vi "strip settings file.vi"(0 "strip array in":string[][](array[string])) -> (1 "time array":timestamp[](array[timestamp]), 2 "settings array out":string[][](array[string]), 3 "timer graph":cluster{cluster{timestamp, dbl}[]}[](graph), 4 "Xscalemax":dbl, 5 "cursor position":dbl, 6 "Xscle min":dbl)   [LabVIEW 2018]
panel:
  out "sec":string
  out "m":string
  out "h":string
  out "DeltaT?":bool
  out "subarray":string[](array[string])
  out "concatenated time string 2":string
  out "function 2":string
  out "cluster 2":T1
  out "strip array 3":string[](array[string])
  out "array of clusters 2":cluster{cluster{timestamp, dbl}[]}[](array[cluster])
  out "cluster":T1
  out "plight":i32=1
  out "mlight":i32=1
  out "function":string
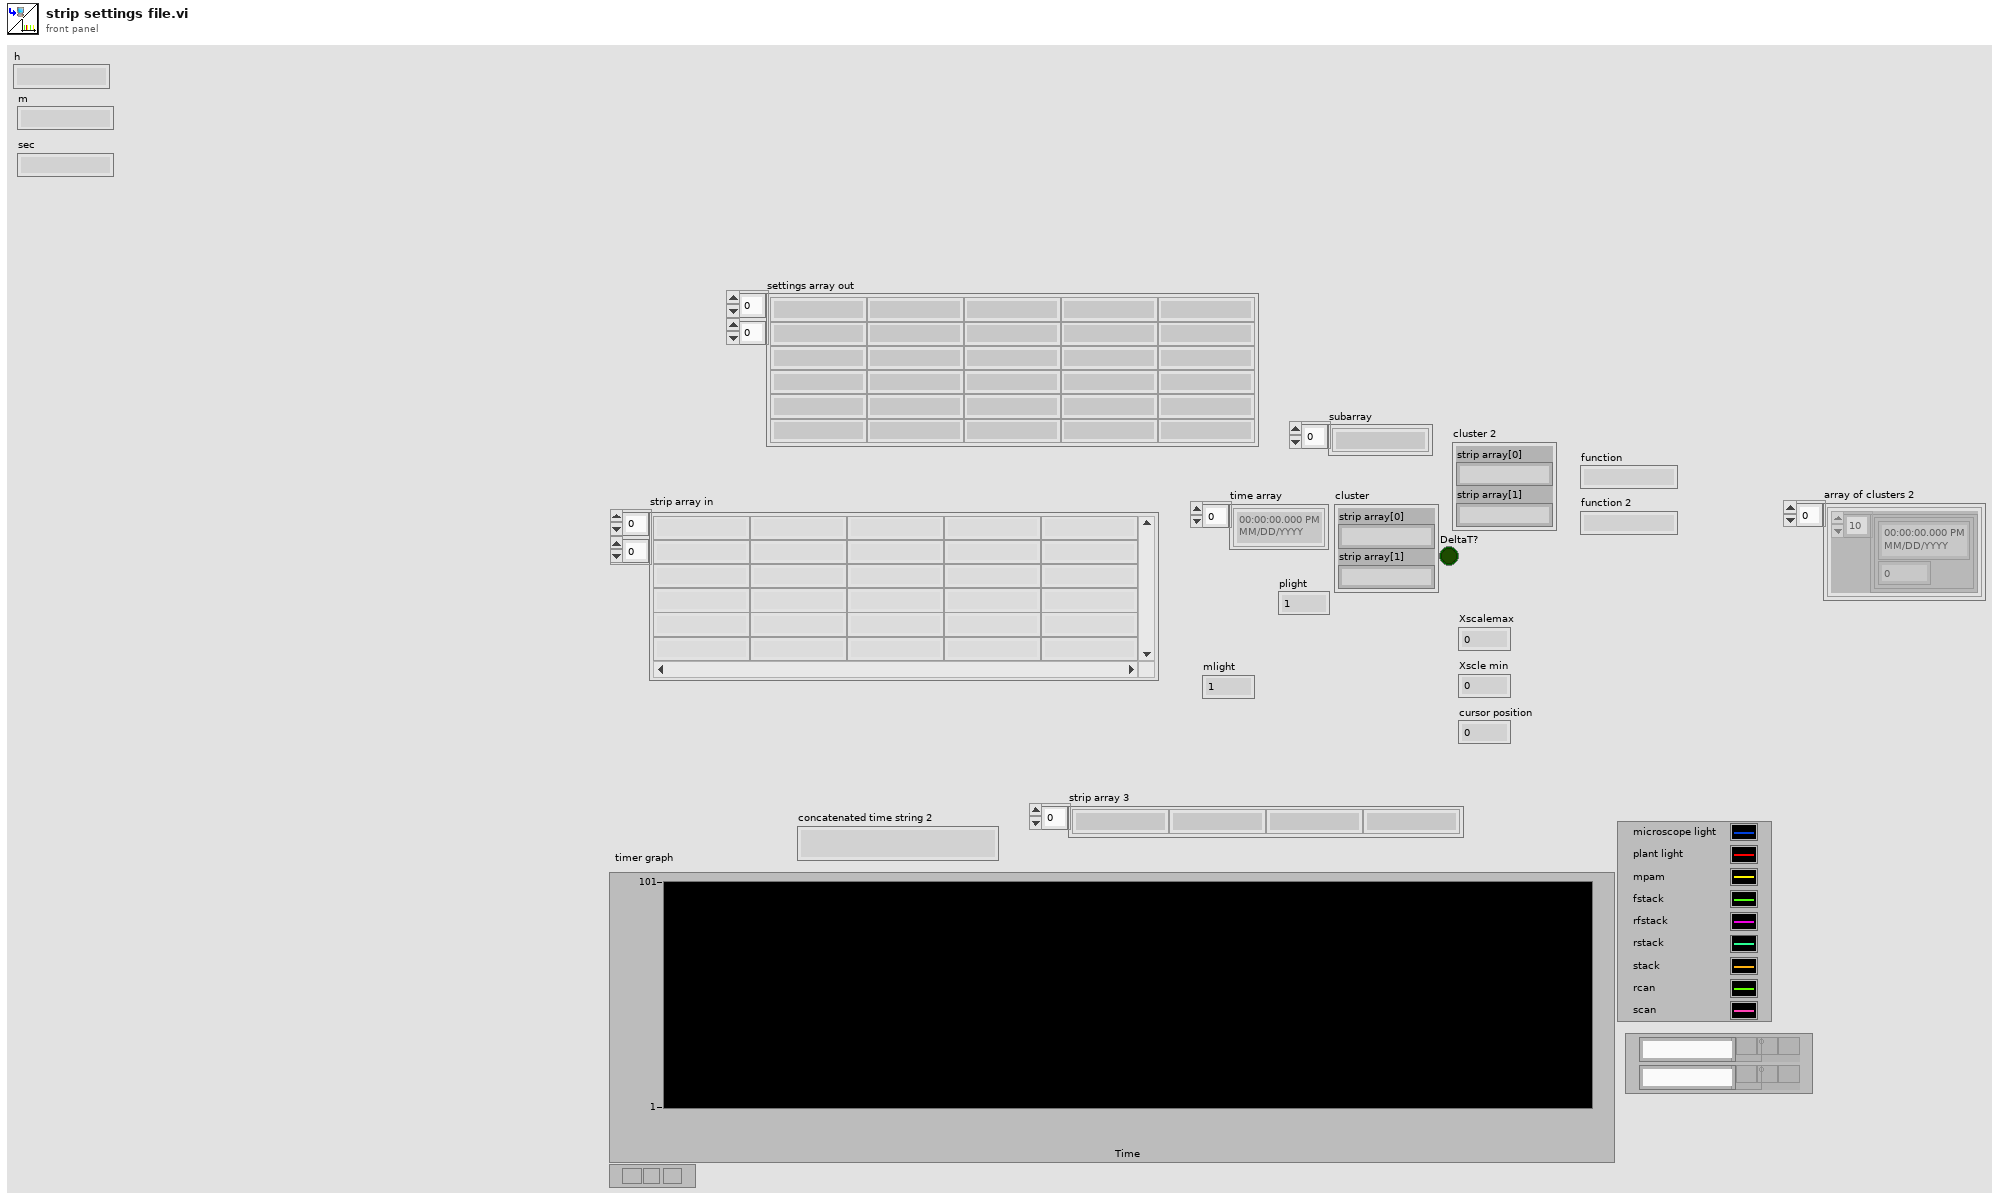
[diagram p1: front panel]
types:
  T1 = cluster{"strip array[0]":string, "strip array[1]":string}
  T2 = cluster{"strip array in[0]":string, "strip array in[1]":string}
  T3 = cluster{"strip array in[0]":string, "strip array in[1]":string, "strip array in[2]":string, "strip array in[3]":string, "strip array in[4]":string, "strip array in[5]":string}
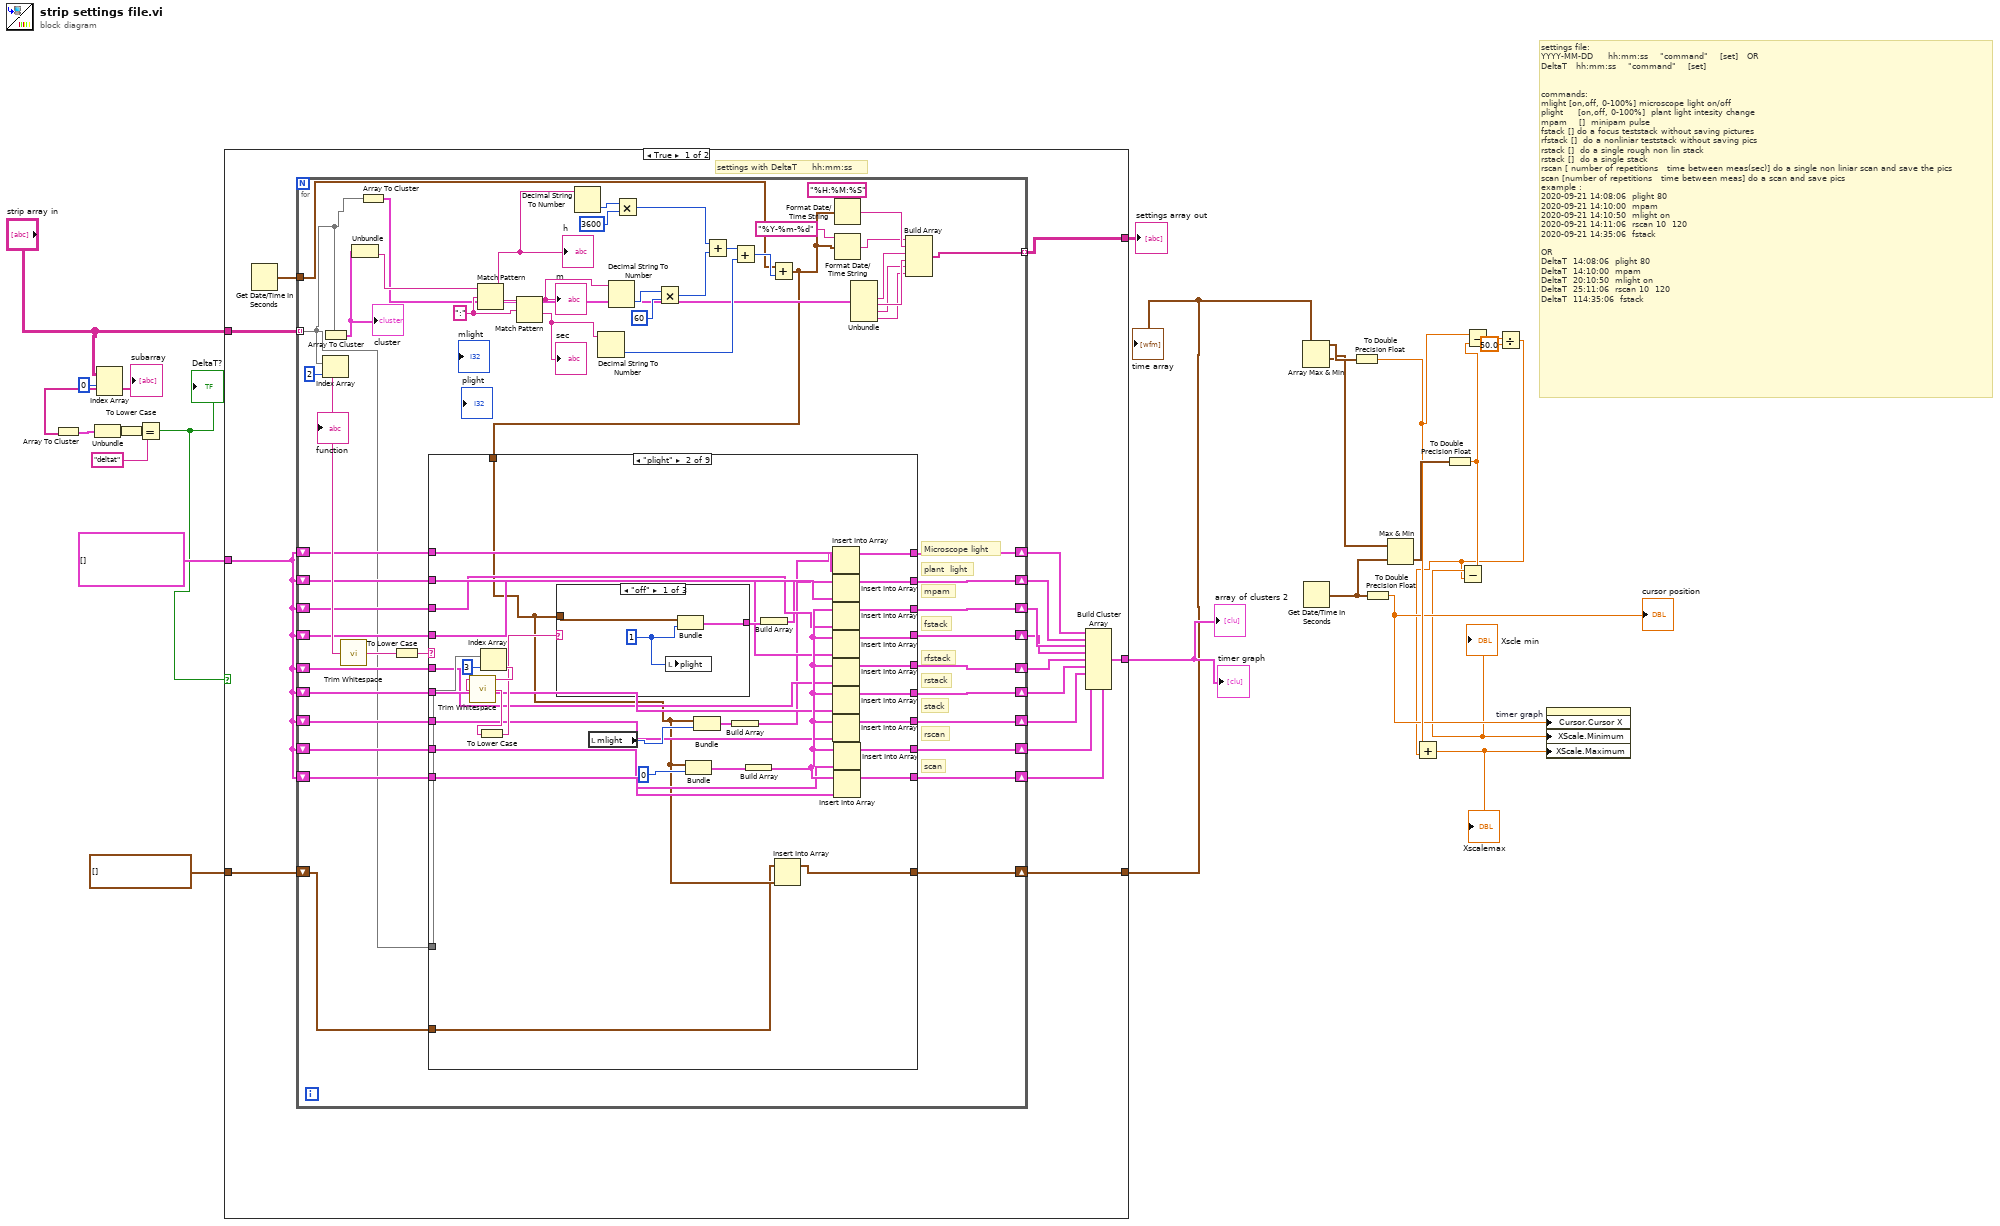
[diagram p0: block diagram]
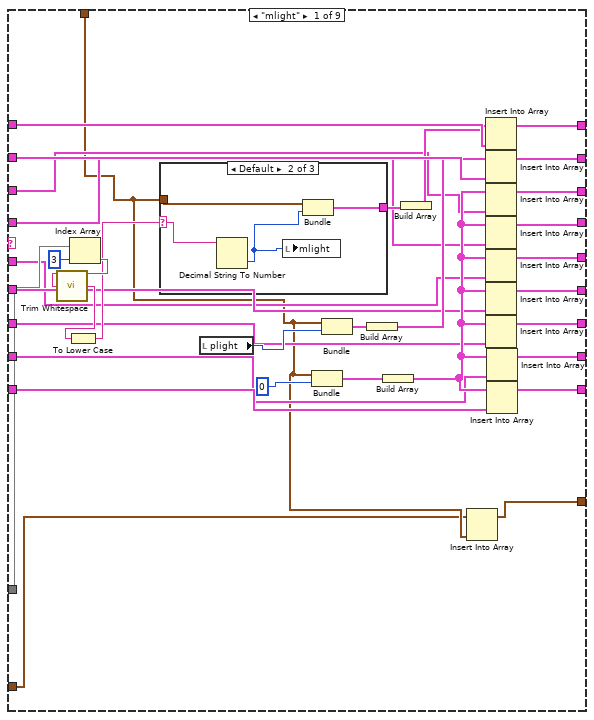
[diagram p2: hidden frame]
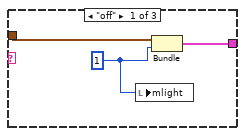
[diagram p3: hidden frame]
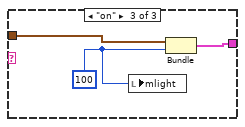
[diagram p4: hidden frame]
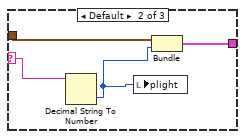
[diagram p5: hidden frame]
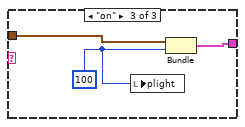
[diagram p6: hidden frame]
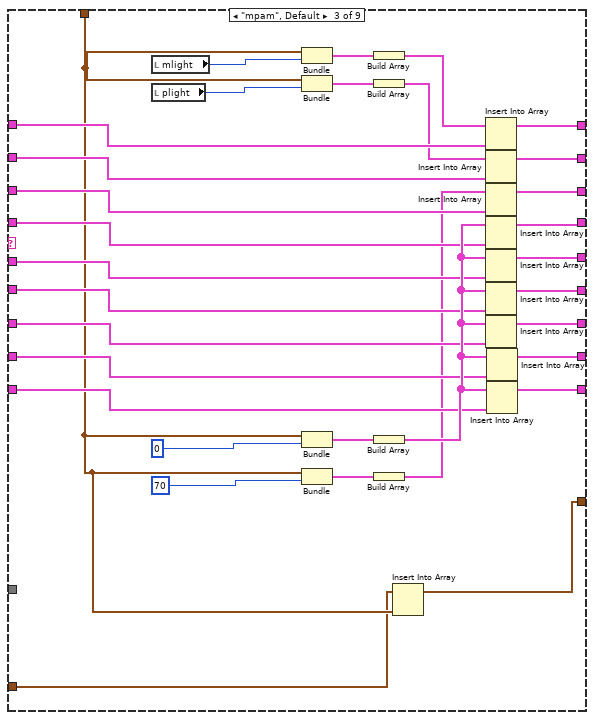
[diagram p7: hidden frame]
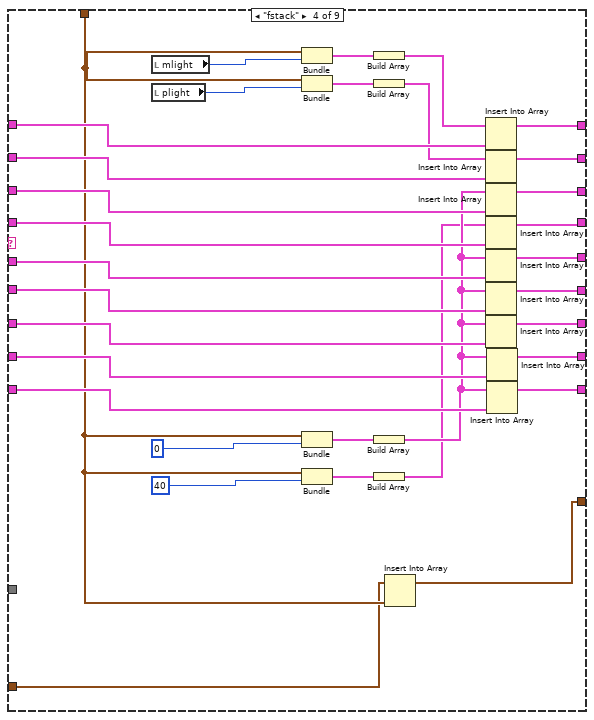
[diagram p8: hidden frame]
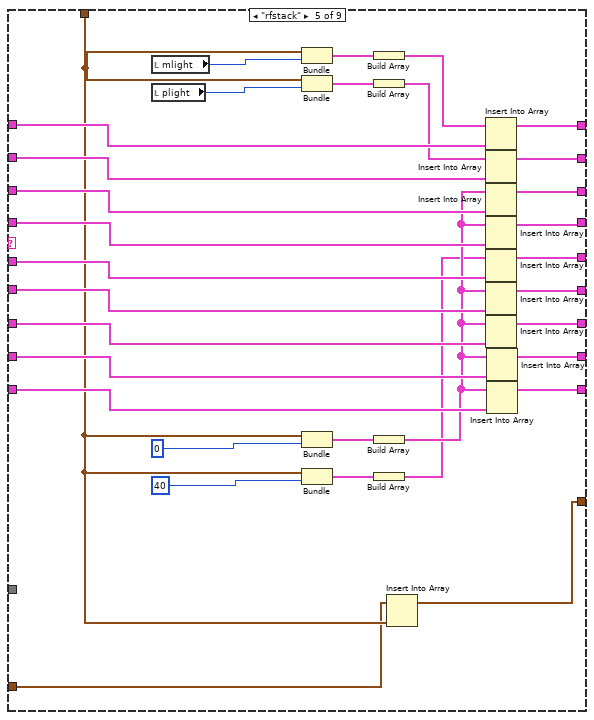
[diagram p9: hidden frame]
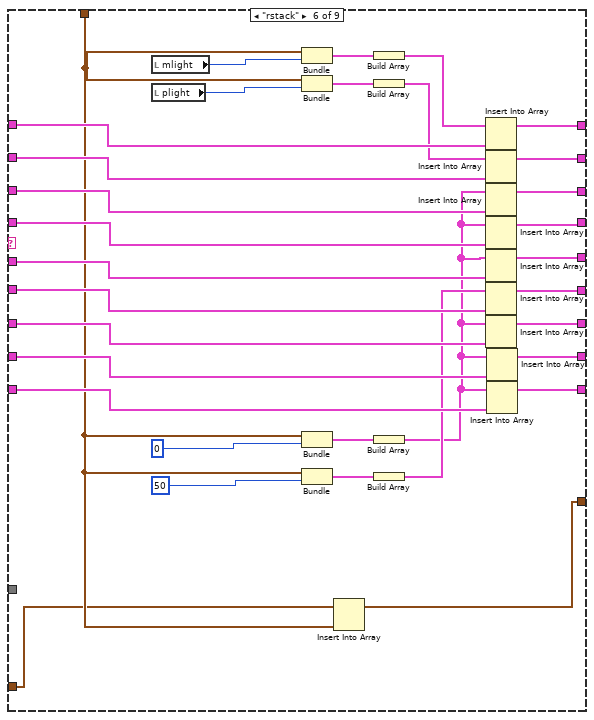
[diagram p10: hidden frame]
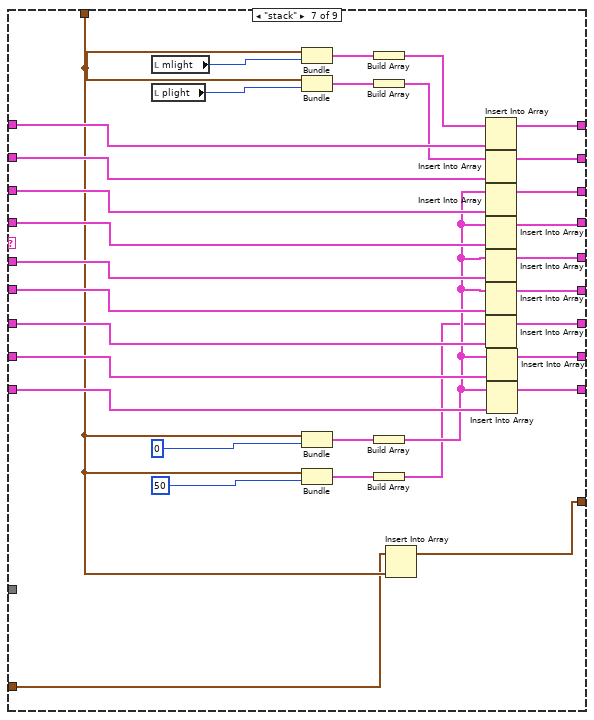
[diagram p11: hidden frame]
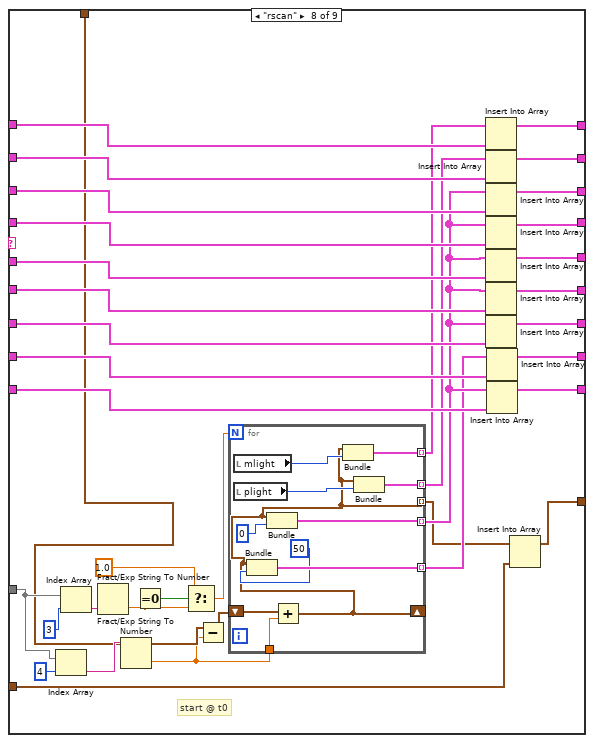
[diagram p12: hidden frame]
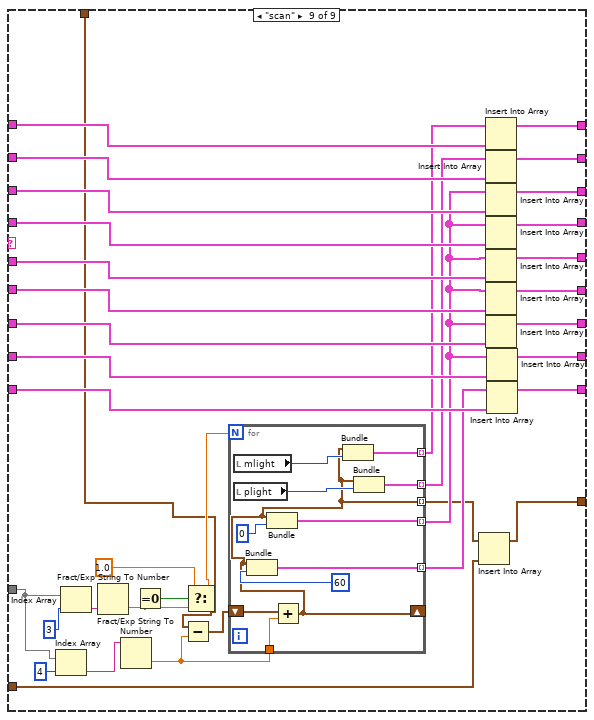
[diagram p13: hidden frame]
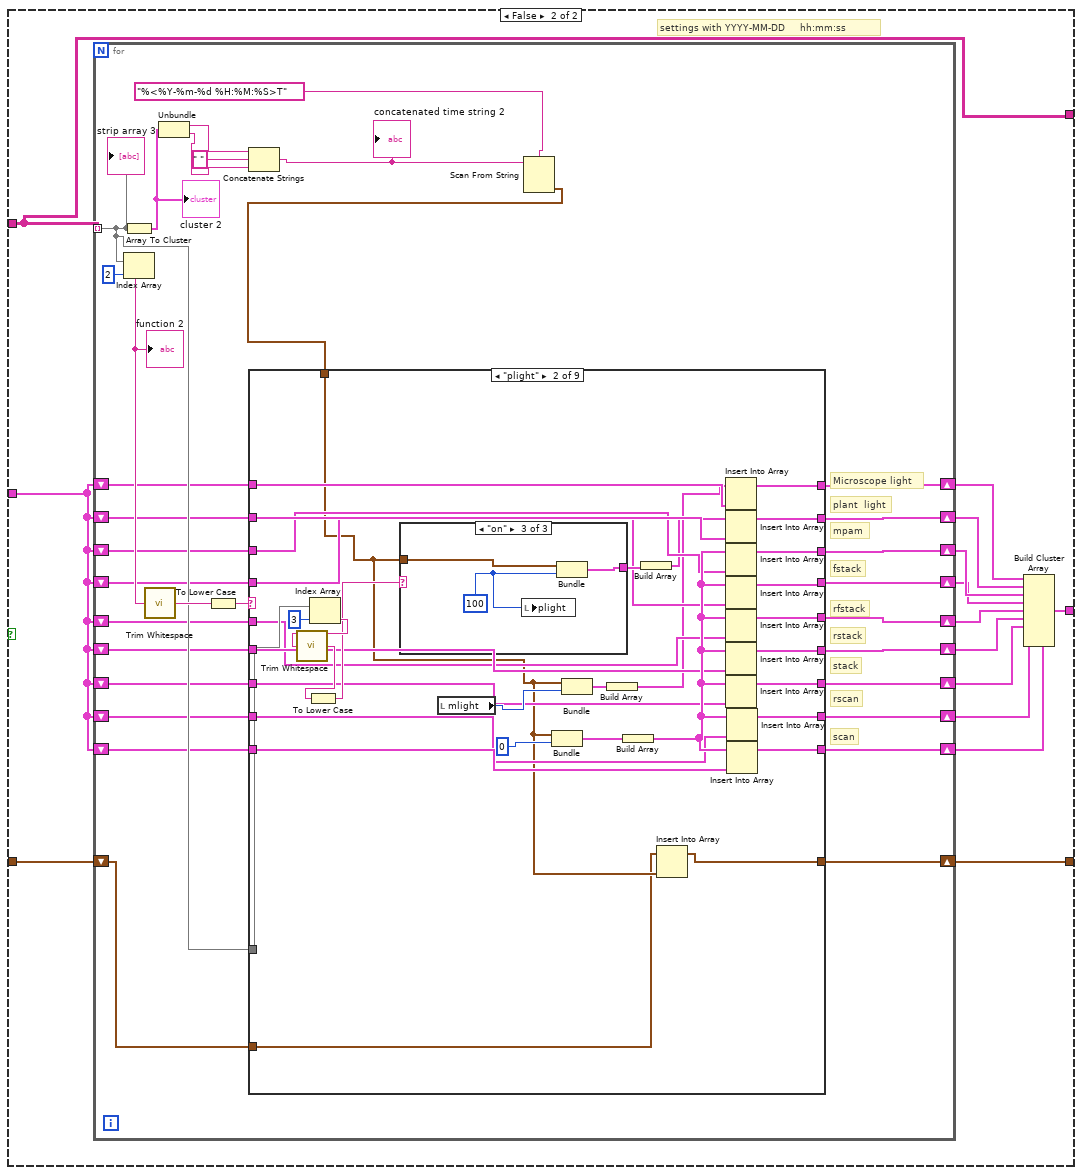
[diagram p14: hidden frame]
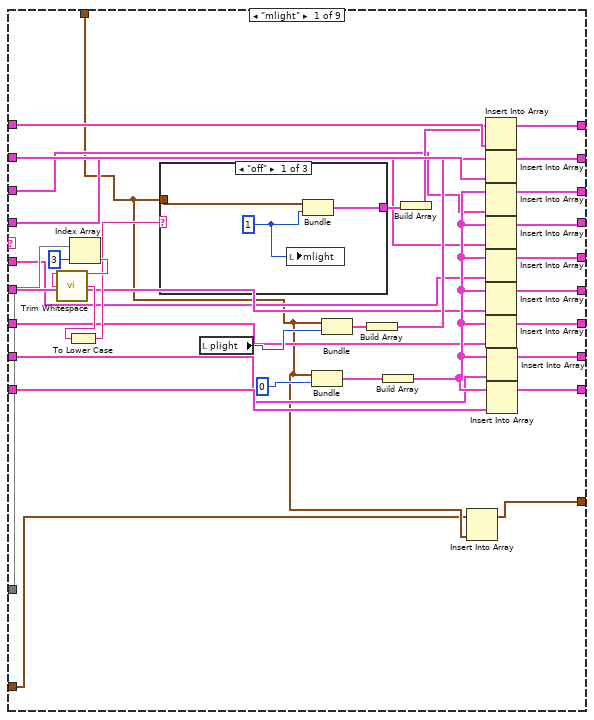
[diagram p15: hidden frame]
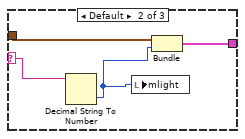
[diagram p16: hidden frame]
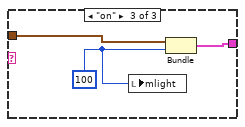
[diagram p17: hidden frame]
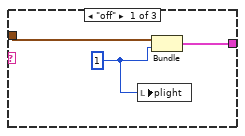
[diagram p18: hidden frame]
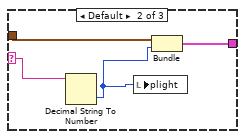
[diagram p19: hidden frame]
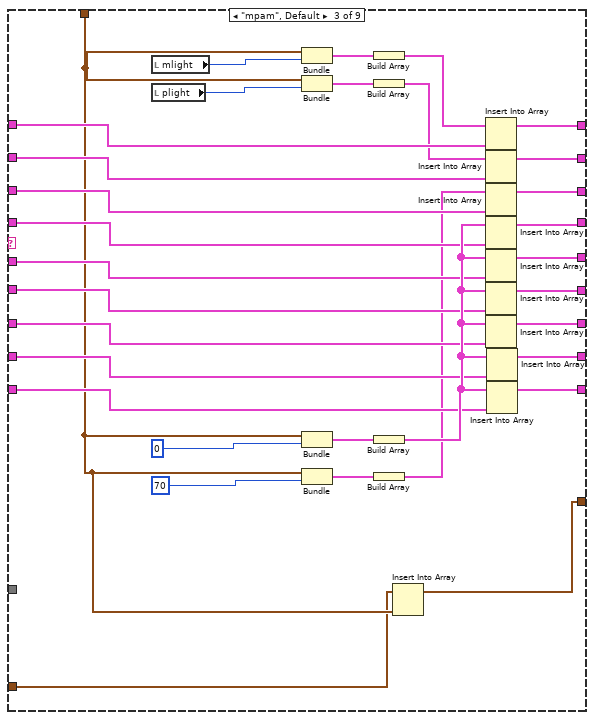
[diagram p20: hidden frame]
diagram:
  # "settings file: \nYYYY-MM-DD\t    hh:mm:ss    \"command\"    [set]   OR\nDeltaT   hh:mm:ss    \"command\"    [set]\n\n\ncommands:\nmlight [on,off, 0-100%] microscope light on/off\nplight     [on,off, 0-100%]  plant light intesity change\nmpam    []  minipam pulse \nfstack [] do a focus teststack without saving pictures\nrfstack []  do a nonliniar teststack without saving pics\nrstack []  do a single rough non lin stack\nrstack []  do a single stack\nrscan [ number of repetitions   time between meas(sec)] do a single non liniar scan and save the pics \nscan [number of repetitions   time between meas] do a scan and save pics\nexample :\n2020-09-21\t14:08:06\t plight\t80\n2020-09-21\t14:10:00\t mpam\n2020-09-21\t14:10:50  mlight on \n2020-09-21\t14:11:06\t rscan 10  120\n2020-09-21\t14:35:06  fstack\n\nOR\nDeltaT\t 14:08:06\t plight\t80\nDeltaT\t 14:10:00\t mpam\nDeltaT\t\t20:10:50  mlight on \nDeltaT\t 25:11:06\t rscan 10  120\nDeltaT\t\t114:35:06  fstack"
  n1 = Index Array(array="strip array in", index (row)=0) -> (element=w7:string[])  [unwired: 1 in]
  "subarray" <- w7
  n2 = Array To Cluster(array=w7) -> (cluster=w6:T2)
  n3 = Unbundle(w6) -> ("strip array in[0]"=w4:string)  [unwired: 1 out]
  n4 = To Lower Case(string=w4) -> (all lower case string=w3:string)
  n5 = Equal?(x=w3, y="deltat") -> (x = y?=w2:bool)
  "DeltaT?" <- w2
  n6 = case shown="True" w2 {
    tunnel: "strip array in" -> [w36 w444]
    tunnel: cluster{timestamp, dbl}[] [] -> [w32 w449]
    tunnel: [w30 w447] -> w12
    tunnel: timestamp[] [] -> [w29 w446]
    tunnel: [w28 w445] -> w10
    tunnel: [w26 w444] -> w1
    frame True {
      # "settings with DeltaT\t    hh:mm:ss"
      n7 = Get Date/Time In Seconds() -> (seconds since 1Jan1904=w27:timestamp)
      n8 = for {
        tunnel: w36 -> [w53] mode=indexing
        shift-right: [w89] -> w31
        shift-left: w32 -> [w79]
        shift-right: [w88] -> w41
        shift-left: w32 -> [w80]
        shift-right: [w87] -> w40
        shift-left: w32 -> [w72]
        shift-right: [w86] -> w39
        shift-left: w32 -> [w73]
        shift-right: [w85] -> w38
        shift-left: w32 -> [w74]
        shift-right: [w84] -> w37
        shift-left: w32 -> [w75]
        shift-right: [w83] -> w35
        shift-left: w32 -> [w76]
        shift-right: [w82] -> w34
        shift-left: w32 -> [w77]
        shift-right: [w81] -> w33
        shift-left: w32 -> [w78]
        shift-right: [w71] -> w28
        shift-left: w29 -> [w70]
        tunnel: w27 -> [w54]
        tunnel: [w47] -> w26 mode=indexing
        w68 = ":" ("regular expression")
        # "scan"
        # "rscan"
        # "stack"
        # "rstack"
        # "rfstack"
        # "fstack"
        # "mpam"
        # "plant  light"
        # "Microscope light"
        n9 = Array To Cluster(array=w53) -> (cluster=w94:T2)
        "cluster" <- w94
        n10 = Index Array(array=w53, index=2) -> (element=w92:string)
        "function" <- w92
        n11 = call <vilib>:"Trim Whitespace.vi"("string"=w92) -> ("trimmed string"=w91:string)  [unwired: 1 in]
        n12 = Unbundle(w94) -> ("strip array in[1]"=w56:string)  [unwired: 1 out]
        n13 = Array To Cluster(array=w53) -> (cluster=w52:T3)
        n14 = To Lower Case(string=w91) -> (all lower case string=w90:string)
        n15 = Match Pattern(string=w56, regular expression=w68) -> (before substring=w67:string, after substring=w69:string)  [unwired: 1 in, 2 out]
        "h" <- w67
        n16 = Match Pattern(string=w69, regular expression=w68) -> (before substring=w66:string, after substring=w65:string)  [unwired: 1 in, 2 out]
        "m" <- w66
        "sec" <- w65
        n17 = Decimal String To Number(string=w67) -> (number=w64:i32)  [unwired: 2 in, 1 out]
        n18 = Decimal String To Number(string=w65) -> (number=w58:i32)  [unwired: 2 in, 1 out]
        n19 = Decimal String To Number(string=w66) -> (number=w57:i32)  [unwired: 2 in, 1 out]
        n20 = Multiply(x=w64, y=3600) -> (x*y=w61:i32)
        n21 = Multiply(x=w57, y=60) -> (x*y=w60:i32)
        n22 = Add(x=w61, y=w60) -> (x+y=w59:i32)
        n23 = Add(x=w59, y=w58) -> (x+y=w55:i32)
        n24 = Add(x=w54, y=w55) -> (x+y=w43:timestamp)
        n25 = case shown="\"plight\"" w90 {
          tunnel: w53 -> [w128 w172 _ _ _ _ _ w359 w406]
          tunnel: [w113 w159 w208 w241 w274 w307 w340 w380 w428] -> w87
          tunnel: w43 -> [w96 w140 w184 w217 w250 w283 w316 w350 w397]
          tunnel: [w117 w162 w210 w243 w276 w309 w342 w382 w430] -> w89
          tunnel: [w121 w165 w213 w246 w279 w312 w345 w384 w432] -> w88
          tunnel: [w112 w158 w207 w240 w273 w306 w339 w379 w427] -> w86
          tunnel: [w111 w157 w206 w239 w272 w305 w338 w378 w426] -> w85
          tunnel: [w110 w156 w205 w238 w271 w304 w337 w377 w425] -> w84
          tunnel: [w109 w155 w204 w237 w270 w303 w336 w376 w424] -> w83
          tunnel: [w108 w154 w203 w236 w269 w302 w335 w375 w423] -> w82
          tunnel: [w107 w153 w202 w235 w268 w301 w334 w374 w422] -> w81
          tunnel: w80 -> [w120 w164 w212 w245 w278 w311 w344 w383 w431]
          tunnel: w79 -> [w116 w161 w209 w242 w275 w308 w341 w381 w429]
          tunnel: w78 -> [w104 w150 w199 w233 w266 w299 w332 w373 w421]
          tunnel: w77 -> [w103 w149 w198 w232 w265 w298 w331 w372 w420]
          tunnel: w76 -> [w102 w148 w197 w231 w264 w297 w330 w371 w419]
          tunnel: w75 -> [w101 w147 w196 w230 w263 w296 w329 w370 w418]
          tunnel: w74 -> [w100 w146 w195 w229 w262 w295 w328 w369 w417]
          tunnel: w73 -> [w99 w145 w194 w228 w261 w294 w327 w368 w416]
          tunnel: w72 -> [w98 w144 w193 w227 w260 w293 w326 w367 w415]
          tunnel: [w97 w141 w185 w218 w251 w284 w317 w354 w401] -> w71
          tunnel: w70 -> [w95 w139 w183 w216 w249 w282 w315 w353 w400]
          frame "mlight" {
            n26 = Index Array(array=w128, index=3) -> (element=w126:string)
            n27 = call <vilib>:"Trim Whitespace.vi"("string"=w126) -> ("trimmed string"=w125:string)  [unwired: 1 in]
            n28 = To Lower Case(string=w125) -> (all lower case string=w124:string)
            n29 = case shown="Default" w124 {
              selector: w124 -> [_ w134 _]
              tunnel: w96 -> [w131 w135 w138]
              tunnel: [w130 w133 w137] -> w115
              frame "off" {
                w129 = 1
                n30 = local write "mlight"(w129) -> ()
                n31 = Bundle(w131, w129) -> (w130:cluster{timestamp, i32})  [unwired: 1 in]
              }
              frame Default {
                n32 = Decimal String To Number(string=w134) -> (number=w132:i32)  [unwired: 2 in, 1 out]
                n33 = local write "mlight"(w132) -> ()
                n34 = Bundle(w135, w132) -> (w133:cluster{timestamp, i32})  [unwired: 1 in]
              }
              frame "on" {
                w136 = 100
                n35 = local write "mlight"(w136) -> ()
                n36 = Bundle(w138, w136) -> (w137:cluster{timestamp, i32})  [unwired: 1 in]
              }
            }
            n37 = local read "plight"() -> (w123:i32)
            n38 = Bundle(w96, 0) -> (w106:cluster{timestamp, i32})  [unwired: 1 in]
            n39 = Bundle(w96, "plight"=w123) -> (w119:cluster{timestamp, "plight":i32})  [unwired: 1 in]
            n40 = Build Array(w119) -> (w118:cluster{timestamp, "plight":i32}[])
            n41 = Build Array(w106) -> (w105:cluster{timestamp, i32}[])
            n42 = Build Array(w115) -> (w114:cluster{timestamp, i32}[])
            n43 = Insert Into Array(array=w95, new element=w96) -> (w97:timestamp[])  [unwired: 1 in]
            n44 = Insert Into Array(array=w114, new element=w116) -> (w117:cluster{timestamp, i32}[])  [unwired: 1 in]
            n45 = Insert Into Array(array=w118, new element=w120) -> (w121:cluster{timestamp, "plight":i32}[])  [unwired: 1 in]
            n46 = Insert Into Array(array=w105, new element=w98) -> (w113:cluster{timestamp, i32}[])  [unwired: 1 in]
            n47 = Insert Into Array(array=w105, new element=w99) -> (w112:cluster{timestamp, i32}[])  [unwired: 1 in]
            n48 = Insert Into Array(array=w105, new element=w100) -> (w111:cluster{timestamp, i32}[])  [unwired: 1 in]
            n49 = Insert Into Array(array=w105, new element=w101) -> (w110:cluster{timestamp, i32}[])  [unwired: 1 in]
            n50 = Insert Into Array(array=w105, new element=w102) -> (w109:cluster{timestamp, i32}[])  [unwired: 1 in]
            n51 = Insert Into Array(array=w105, new element=w103) -> (w108:cluster{timestamp, i32}[])  [unwired: 1 in]
            n52 = Insert Into Array(array=w105, new element=w104) -> (w107:cluster{timestamp, i32}[])  [unwired: 1 in]
          }
          frame "plight" {
            n53 = Index Array(array=w172, index=3) -> (element=w170:string)
            n54 = call <vilib>:"Trim Whitespace.vi"("string"=w170) -> ("trimmed string"=w169:string)  [unwired: 1 in]
            n55 = To Lower Case(string=w169) -> (all lower case string=w168:string)
            n56 = case shown="\"off\"" w168 {
              selector: w168 -> [_ w178 _]
              tunnel: w140 -> [w175 w179 w182]
              tunnel: [w174 w177 w181] -> w160
              frame "off" {
                w173 = 1
                n57 = local write "plight"(w173) -> ()
                n58 = Bundle(w175, w173) -> (w174:cluster{timestamp, i32})  [unwired: 1 in]
              }
              frame Default {
                n59 = Decimal String To Number(string=w178) -> (number=w176:i32)  [unwired: 2 in, 1 out]
                n60 = local write "plight"(w176) -> ()
                n61 = Bundle(w179, w176) -> (w177:cluster{timestamp, i32})  [unwired: 1 in]
              }
              frame "on" {
                w180 = 100
                n62 = local write "plight"(w180) -> ()
                n63 = Bundle(w182, w180) -> (w181:cluster{timestamp, i32})  [unwired: 1 in]
              }
            }
            n64 = local read "mlight"() -> (w167:i32)
            n65 = Bundle(w140, 0) -> (w152:cluster{timestamp, i32})  [unwired: 1 in]
            n66 = Bundle(w140, "mlight"=w167) -> (w163:cluster{timestamp, "mlight":i32})  [unwired: 1 in]
            n67 = Build Array(w163) -> (w143:cluster{timestamp, "mlight":i32}[])
            n68 = Build Array(w152) -> (w151:cluster{timestamp, i32}[])
            n69 = Build Array(w160) -> (w142:cluster{timestamp, i32}[])
            n70 = Insert Into Array(array=w139, new element=w140) -> (w141:timestamp[])  [unwired: 1 in]
            n71 = Insert Into Array(array=w143, new element=w161) -> (w162:cluster{timestamp, "mlight":i32}[])  [unwired: 1 in]
            n72 = Insert Into Array(array=w142, new element=w164) -> (w165:cluster{timestamp, i32}[])  [unwired: 1 in]
            n73 = Insert Into Array(array=w151, new element=w144) -> (w159:cluster{timestamp, i32}[])  [unwired: 1 in]
            n74 = Insert Into Array(array=w151, new element=w145) -> (w158:cluster{timestamp, i32}[])  [unwired: 1 in]
            n75 = Insert Into Array(array=w151, new element=w146) -> (w157:cluster{timestamp, i32}[])  [unwired: 1 in]
            n76 = Insert Into Array(array=w151, new element=w147) -> (w156:cluster{timestamp, i32}[])  [unwired: 1 in]
            n77 = Insert Into Array(array=w151, new element=w148) -> (w155:cluster{timestamp, i32}[])  [unwired: 1 in]
            n78 = Insert Into Array(array=w151, new element=w149) -> (w154:cluster{timestamp, i32}[])  [unwired: 1 in]
            n79 = Insert Into Array(array=w151, new element=w150) -> (w153:cluster{timestamp, i32}[])  [unwired: 1 in]
          }
          frame "mpam", Default {
            n80 = local read "mlight"() -> (w215:i32)
            n81 = local read "plight"() -> (w190:i32)
            n82 = Bundle(w184, "mlight"=w215) -> (w211:cluster{timestamp, "mlight":i32})  [unwired: 1 in]
            n83 = Bundle(w184, "plight"=w190) -> (w188:cluster{timestamp, "plight":i32})  [unwired: 1 in]
            n84 = Bundle(w184, 0) -> (w201:cluster{timestamp, i32})  [unwired: 1 in]
            n85 = Bundle(w184, 70) -> (w187:cluster{timestamp, i32})  [unwired: 1 in]
            n86 = Build Array(w211) -> (w192:cluster{timestamp, "mlight":i32}[])
            n87 = Build Array(w188) -> (w191:cluster{timestamp, "plight":i32}[])
            n88 = Build Array(w201) -> (w200:cluster{timestamp, i32}[])
            n89 = Build Array(w187) -> (w186:cluster{timestamp, i32}[])
            n90 = Insert Into Array(array=w183, new element=w184) -> (w185:timestamp[])  [unwired: 1 in]
            n91 = Insert Into Array(array=w192, new element=w209) -> (w210:cluster{timestamp, "mlight":i32}[])  [unwired: 1 in]
            n92 = Insert Into Array(array=w191, new element=w212) -> (w213:cluster{timestamp, "plight":i32}[])  [unwired: 1 in]
            n93 = Insert Into Array(array=w186, new element=w193) -> (w208:cluster{timestamp, i32}[])  [unwired: 1 in]
            n94 = Insert Into Array(array=w200, new element=w194) -> (w207:cluster{timestamp, i32}[])  [unwired: 1 in]
            n95 = Insert Into Array(array=w200, new element=w195) -> (w206:cluster{timestamp, i32}[])  [unwired: 1 in]
            n96 = Insert Into Array(array=w200, new element=w196) -> (w205:cluster{timestamp, i32}[])  [unwired: 1 in]
            n97 = Insert Into Array(array=w200, new element=w197) -> (w204:cluster{timestamp, i32}[])  [unwired: 1 in]
            n98 = Insert Into Array(array=w200, new element=w198) -> (w203:cluster{timestamp, i32}[])  [unwired: 1 in]
            n99 = Insert Into Array(array=w200, new element=w199) -> (w202:cluster{timestamp, i32}[])  [unwired: 1 in]
          }
          frame "fstack" {
            n100 = local read "mlight"() -> (w248:i32)
            n101 = local read "plight"() -> (w224:i32)
            n102 = Bundle(w217, "mlight"=w248) -> (w244:cluster{timestamp, "mlight":i32})  [unwired: 1 in]
            n103 = Bundle(w217, "plight"=w224) -> (w222:cluster{timestamp, "plight":i32})  [unwired: 1 in]
            n104 = Bundle(w217, 0) -> (w234:cluster{timestamp, i32})  [unwired: 1 in]
            n105 = Bundle(w217, 40) -> (w221:cluster{timestamp, i32})  [unwired: 1 in]
            n106 = Build Array(w244) -> (w226:cluster{timestamp, "mlight":i32}[])
            n107 = Build Array(w222) -> (w225:cluster{timestamp, "plight":i32}[])
            n108 = Build Array(w234) -> (w220:cluster{timestamp, i32}[])
            n109 = Build Array(w221) -> (w219:cluster{timestamp, i32}[])
            n110 = Insert Into Array(array=w216, new element=w217) -> (w218:timestamp[])  [unwired: 1 in]
            n111 = Insert Into Array(array=w226, new element=w242) -> (w243:cluster{timestamp, "mlight":i32}[])  [unwired: 1 in]
            n112 = Insert Into Array(array=w225, new element=w245) -> (w246:cluster{timestamp, "plight":i32}[])  [unwired: 1 in]
            n113 = Insert Into Array(array=w220, new element=w227) -> (w241:cluster{timestamp, i32}[])  [unwired: 1 in]
            n114 = Insert Into Array(array=w219, new element=w228) -> (w240:cluster{timestamp, i32}[])  [unwired: 1 in]
            n115 = Insert Into Array(array=w220, new element=w229) -> (w239:cluster{timestamp, i32}[])  [unwired: 1 in]
            n116 = Insert Into Array(array=w220, new element=w230) -> (w238:cluster{timestamp, i32}[])  [unwired: 1 in]
            n117 = Insert Into Array(array=w220, new element=w231) -> (w237:cluster{timestamp, i32}[])  [unwired: 1 in]
            n118 = Insert Into Array(array=w220, new element=w232) -> (w236:cluster{timestamp, i32}[])  [unwired: 1 in]
            n119 = Insert Into Array(array=w220, new element=w233) -> (w235:cluster{timestamp, i32}[])  [unwired: 1 in]
          }
          frame "rfstack" {
            n120 = local read "mlight"() -> (w281:i32)
            n121 = local read "plight"() -> (w257:i32)
            n122 = Bundle(w250, "mlight"=w281) -> (w277:cluster{timestamp, "mlight":i32})  [unwired: 1 in]
            n123 = Bundle(w250, "plight"=w257) -> (w255:cluster{timestamp, "plight":i32})  [unwired: 1 in]
            n124 = Bundle(w250, 0) -> (w267:cluster{timestamp, i32})  [unwired: 1 in]
            n125 = Bundle(w250, 40) -> (w254:cluster{timestamp, i32})  [unwired: 1 in]
            n126 = Build Array(w277) -> (w259:cluster{timestamp, "mlight":i32}[])
            n127 = Build Array(w255) -> (w258:cluster{timestamp, "plight":i32}[])
            n128 = Build Array(w267) -> (w253:cluster{timestamp, i32}[])
            n129 = Build Array(w254) -> (w252:cluster{timestamp, i32}[])
            n130 = Insert Into Array(array=w249, new element=w250) -> (w251:timestamp[])  [unwired: 1 in]
            n131 = Insert Into Array(array=w259, new element=w275) -> (w276:cluster{timestamp, "mlight":i32}[])  [unwired: 1 in]
            n132 = Insert Into Array(array=w258, new element=w278) -> (w279:cluster{timestamp, "plight":i32}[])  [unwired: 1 in]
            n133 = Insert Into Array(array=w253, new element=w260) -> (w274:cluster{timestamp, i32}[])  [unwired: 1 in]
            n134 = Insert Into Array(array=w253, new element=w261) -> (w273:cluster{timestamp, i32}[])  [unwired: 1 in]
            n135 = Insert Into Array(array=w252, new element=w262) -> (w272:cluster{timestamp, i32}[])  [unwired: 1 in]
            n136 = Insert Into Array(array=w253, new element=w263) -> (w271:cluster{timestamp, i32}[])  [unwired: 1 in]
            n137 = Insert Into Array(array=w253, new element=w264) -> (w270:cluster{timestamp, i32}[])  [unwired: 1 in]
            n138 = Insert Into Array(array=w253, new element=w265) -> (w269:cluster{timestamp, i32}[])  [unwired: 1 in]
            n139 = Insert Into Array(array=w253, new element=w266) -> (w268:cluster{timestamp, i32}[])  [unwired: 1 in]
          }
          frame "rstack" {
            n140 = local read "mlight"() -> (w314:i32)
            n141 = local read "plight"() -> (w290:i32)
            n142 = Bundle(w283, "mlight"=w314) -> (w310:cluster{timestamp, "mlight":i32})  [unwired: 1 in]
            n143 = Bundle(w283, "plight"=w290) -> (w288:cluster{timestamp, "plight":i32})  [unwired: 1 in]
            n144 = Bundle(w283, 0) -> (w300:cluster{timestamp, i32})  [unwired: 1 in]
            n145 = Bundle(w283, 50) -> (w287:cluster{timestamp, i32})  [unwired: 1 in]
            n146 = Insert Into Array(array=w282, new element=w283) -> (w284:timestamp[])  [unwired: 1 in]
            n147 = Build Array(w310) -> (w292:cluster{timestamp, "mlight":i32}[])
            n148 = Build Array(w288) -> (w291:cluster{timestamp, "plight":i32}[])
            n149 = Build Array(w300) -> (w285:cluster{timestamp, i32}[])
            n150 = Build Array(w287) -> (w286:cluster{timestamp, i32}[])
            n151 = Insert Into Array(array=w292, new element=w308) -> (w309:cluster{timestamp, "mlight":i32}[])  [unwired: 1 in]
            n152 = Insert Into Array(array=w291, new element=w311) -> (w312:cluster{timestamp, "plight":i32}[])  [unwired: 1 in]
            n153 = Insert Into Array(array=w285, new element=w293) -> (w307:cluster{timestamp, i32}[])  [unwired: 1 in]
            n154 = Insert Into Array(array=w285, new element=w294) -> (w306:cluster{timestamp, i32}[])  [unwired: 1 in]
            n155 = Insert Into Array(array=w285, new element=w295) -> (w305:cluster{timestamp, i32}[])  [unwired: 1 in]
            n156 = Insert Into Array(array=w286, new element=w296) -> (w304:cluster{timestamp, i32}[])  [unwired: 1 in]
            n157 = Insert Into Array(array=w285, new element=w297) -> (w303:cluster{timestamp, i32}[])  [unwired: 1 in]
            n158 = Insert Into Array(array=w285, new element=w298) -> (w302:cluster{timestamp, i32}[])  [unwired: 1 in]
            n159 = Insert Into Array(array=w285, new element=w299) -> (w301:cluster{timestamp, i32}[])  [unwired: 1 in]
          }
          frame "stack" {
            n160 = local read "mlight"() -> (w347:i32)
            n161 = local read "plight"() -> (w323:i32)
            n162 = Bundle(w316, "mlight"=w347) -> (w343:cluster{timestamp, "mlight":i32})  [unwired: 1 in]
            n163 = Bundle(w316, "plight"=w323) -> (w321:cluster{timestamp, "plight":i32})  [unwired: 1 in]
            n164 = Bundle(w316, 0) -> (w333:cluster{timestamp, i32})  [unwired: 1 in]
            n165 = Bundle(w316, 50) -> (w320:cluster{timestamp, i32})  [unwired: 1 in]
            n166 = Build Array(w343) -> (w325:cluster{timestamp, "mlight":i32}[])
            n167 = Build Array(w321) -> (w324:cluster{timestamp, "plight":i32}[])
            n168 = Build Array(w333) -> (w319:cluster{timestamp, i32}[])
            n169 = Build Array(w320) -> (w318:cluster{timestamp, i32}[])
            n170 = Insert Into Array(array=w315, new element=w316) -> (w317:timestamp[])  [unwired: 1 in]
            n171 = Insert Into Array(array=w325, new element=w341) -> (w342:cluster{timestamp, "mlight":i32}[])  [unwired: 1 in]
            n172 = Insert Into Array(array=w324, new element=w344) -> (w345:cluster{timestamp, "plight":i32}[])  [unwired: 1 in]
            n173 = Insert Into Array(array=w319, new element=w326) -> (w340:cluster{timestamp, i32}[])  [unwired: 1 in]
            n174 = Insert Into Array(array=w319, new element=w327) -> (w339:cluster{timestamp, i32}[])  [unwired: 1 in]
            n175 = Insert Into Array(array=w319, new element=w328) -> (w338:cluster{timestamp, i32}[])  [unwired: 1 in]
            n176 = Insert Into Array(array=w319, new element=w329) -> (w337:cluster{timestamp, i32}[])  [unwired: 1 in]
            n177 = Insert Into Array(array=w318, new element=w330) -> (w336:cluster{timestamp, i32}[])  [unwired: 1 in]
            n178 = Insert Into Array(array=w319, new element=w331) -> (w335:cluster{timestamp, i32}[])  [unwired: 1 in]
            n179 = Insert Into Array(array=w319, new element=w332) -> (w334:cluster{timestamp, i32}[])  [unwired: 1 in]
          }
          frame "rscan" {
            # "start @ t0"
            n180 = Index Array(array=w359, index=4) -> (element=w363:string)
            n181 = Index Array(array=w359, index=3) -> (element=w365:string)
            n182 = Fract/Exp String To Number(string=w365) -> (number=w362:dbl)  [unwired: 3 in, 1 out]
            n183 = Fract/Exp String To Number(string=w363) -> (number=w348:dbl)  [unwired: 3 in, 1 out]
            n184 = Equal To 0?(x=w362) -> (x = 0?=w361:bool)
            n185 = Select(t=1.0, s=w361, f=w362) -> (s? t:f=w351:dbl)
            n186 = Subtract(x=w350, y=w348) -> (x-y=w349:timestamp)
            n187 = for {
              N: w351 -> [_]
              tunnel: [w395] -> w357 mode=indexing
              tunnel: w348 -> [w394]
              shift-right: [w385] -> _
              shift-left: w349 -> [w393]
              tunnel: [w392] -> w358 mode=indexing
              tunnel: [w388] -> w356 mode=indexing
              tunnel: [w387] -> w355 mode=indexing
              tunnel: [w385] -> w352 mode=indexing
              n188 = local read "mlight"() -> (w389:i32)
              n189 = local read "plight"() -> (w390:i32)
              n190 = Add(x=w393, y=w394) -> (x+y=w385:timestamp)
              n191 = Bundle(w385, 50) -> (w395:cluster{timestamp, i32})  [unwired: 1 in]
              n192 = Bundle(w385, 0) -> (w392:cluster{timestamp, i32})  [unwired: 1 in]
              n193 = Bundle(w385, "mlight"=w389) -> (w388:cluster{timestamp, "mlight":i32})  [unwired: 1 in]
              n194 = Bundle(w385, "plight"=w390) -> (w387:cluster{timestamp, "plight":i32})  [unwired: 1 in]
            }
            n195 = Insert Into Array(array=w356, new element=w381) -> (w382:cluster{timestamp, "mlight":i32}[])  [unwired: 1 in]
            n196 = Insert Into Array(array=w355, new element=w383) -> (w384:cluster{timestamp, "plight":i32}[])  [unwired: 1 in]
            n197 = Insert Into Array(array=w358, new element=w367) -> (w380:cluster{timestamp, i32}[])  [unwired: 1 in]
            n198 = Insert Into Array(array=w358, new element=w368) -> (w379:cluster{timestamp, i32}[])  [unwired: 1 in]
            n199 = Insert Into Array(array=w358, new element=w369) -> (w378:cluster{timestamp, i32}[])  [unwired: 1 in]
            n200 = Insert Into Array(array=w358, new element=w370) -> (w377:cluster{timestamp, i32}[])  [unwired: 1 in]
            n201 = Insert Into Array(array=w358, new element=w371) -> (w376:cluster{timestamp, i32}[])  [unwired: 1 in]
            n202 = Insert Into Array(array=w357, new element=w372) -> (w375:cluster{timestamp, i32}[])  [unwired: 1 in]
            n203 = Insert Into Array(array=w358, new element=w373) -> (w374:cluster{timestamp, i32}[])  [unwired: 1 in]
            n204 = Insert Into Array(array=w352, new element=w353) -> (w354:timestamp[])  [unwired: 1 in]
          }
          frame "scan" {
            n205 = Index Array(array=w406, index=4) -> (element=w411:string)
            n206 = Index Array(array=w406, index=3) -> (element=w413:string)
            n207 = Fract/Exp String To Number(string=w413) -> (number=w410:dbl)  [unwired: 3 in, 1 out]
            n208 = Fract/Exp String To Number(string=w411) -> (number=w396:dbl)  [unwired: 3 in, 1 out]
            n209 = Equal To 0?(x=w410) -> (x = 0?=w409:bool)
            n210 = Subtract(x=w397, y=w396) -> (x-y=w398:timestamp)
            n211 = Select(t=1.0, s=w409, f=w410) -> (s? t:f=w407:dbl)
            n212 = for {
              N: w407 -> [_]
              tunnel: [w443] -> w403 mode=indexing
              tunnel: w396 -> [w442]
              shift-right: [w433] -> _
              shift-left: w398 -> [w441]
              tunnel: [w440] -> w402 mode=indexing
              tunnel: [w436] -> w405 mode=indexing
              tunnel: [w435] -> w404 mode=indexing
              tunnel: [w433] -> w399 mode=indexing
              n213 = local read "mlight"() -> (w437:i32)
              n214 = local read "plight"() -> (w438:i32)
              n215 = Add(x=w441, y=w442) -> (x+y=w433:timestamp)
              n216 = Bundle(w433, 60) -> (w443:cluster{timestamp, i32})  [unwired: 1 in]
              n217 = Bundle(w433, 0) -> (w440:cluster{timestamp, i32})  [unwired: 1 in]
              n218 = Bundle(w433, "mlight"=w437) -> (w436:cluster{timestamp, "mlight":i32})  [unwired: 1 in]
              n219 = Bundle(w433, "plight"=w438) -> (w435:cluster{timestamp, "plight":i32})  [unwired: 1 in]
            }
            n220 = Insert Into Array(array=w399, new element=w400) -> (w401:timestamp[])  [unwired: 1 in]
            n221 = Insert Into Array(array=w405, new element=w429) -> (w430:cluster{timestamp, "mlight":i32}[])  [unwired: 1 in]
            n222 = Insert Into Array(array=w404, new element=w431) -> (w432:cluster{timestamp, "plight":i32}[])  [unwired: 1 in]
            n223 = Insert Into Array(array=w402, new element=w415) -> (w428:cluster{timestamp, i32}[])  [unwired: 1 in]
            n224 = Insert Into Array(array=w402, new element=w416) -> (w427:cluster{timestamp, i32}[])  [unwired: 1 in]
            n225 = Insert Into Array(array=w402, new element=w417) -> (w426:cluster{timestamp, i32}[])  [unwired: 1 in]
            n226 = Insert Into Array(array=w402, new element=w418) -> (w425:cluster{timestamp, i32}[])  [unwired: 1 in]
            n227 = Insert Into Array(array=w402, new element=w419) -> (w424:cluster{timestamp, i32}[])  [unwired: 1 in]
            n228 = Insert Into Array(array=w402, new element=w420) -> (w423:cluster{timestamp, i32}[])  [unwired: 1 in]
            n229 = Insert Into Array(array=w403, new element=w421) -> (w422:cluster{timestamp, i32}[])  [unwired: 1 in]
          }
        }
        n230 = Format Date/Time String(time format string (%c)="%H:%M:%S" ("format string"), seconds (now)=w43) -> (date/time string=w46:string)  [unwired: 1 in]
        n231 = Format Date/Time String(time format string (%c)="%Y-%m-%d" ("format string"), seconds (now)=w43) -> (date/time string=w44:string)  [unwired: 1 in]
        n232 = Unbundle(w52) -> ("strip array in[2]"=w51:string, "strip array in[3]"=w50:string, "strip array in[4]"=w49:string, "strip array in[5]"=w48:string)  [unwired: 2 out]
        n233 = Build Array(w44, w46, w51, w50, w49, w48) -> (w47:string[])
      }
      n234 = Build Cluster Array(w31, w41, w40, w39, w38, w37, w35, w34, w33) -> (w30:cluster{cluster{timestamp, dbl}[]}[])
    }
    frame False {
      # "settings with YYYY-MM-DD\t    hh:mm:ss"
      n235 = for {
        tunnel: w444 -> [w479] mode=indexing
        shift-right: [w477] -> w448
        shift-left: w449 -> [w467]
        shift-right: [w476] -> w457
        shift-left: w449 -> [w468]
        shift-right: [w475] -> w456
        shift-left: w449 -> [w460]
        shift-right: [w474] -> w455
        shift-left: w449 -> [w461]
        shift-right: [w473] -> w454
        shift-left: w449 -> [w462]
        shift-right: [w472] -> w453
        shift-left: w449 -> [w463]
        shift-right: [w471] -> w452
        shift-left: w449 -> [w464]
        shift-right: [w470] -> w451
        shift-left: w449 -> [w465]
        shift-right: [w469] -> w450
        shift-left: w449 -> [w466]
        shift-right: [w459] -> w445
        shift-left: w446 -> [w458]
        # "scan"
        # "rscan"
        # "stack"
        # "rstack"
        # "rfstack"
        # "fstack"
        # "mpam"
        # "plant  light"
        # "Microscope light"
        n236 = Array To Cluster(array=w479) -> (cluster=w484:T2)
        "cluster 2" <- w484
        n237 = Index Array(array=w479, index=2) -> (element=w482:string)
        "function 2" <- w482
        n238 = call <vilib>:"Trim Whitespace.vi"("string"=w482) -> ("trimmed string"=w481:string)  [unwired: 1 in]
        n239 = Unbundle(w484) -> ("strip array in[0]"=w486:string, "strip array in[1]"=w485:string)
        n240 = To Lower Case(string=w481) -> (all lower case string=w480:string)
        n241 = Concatenate Strings(w486, " " ("string"), w485) -> (w489:string)
        "concatenated time string 2" <- w489
        n242 = Scan From String(format string="%<%Y-%m-%d %H:%M:%S>T", input string=w489) -> (output 1=w478:timestamp)  [unwired: 3 in, 3 out]
        n243 = case shown="\"plight\"" w480 {
          tunnel: w479 -> [w523 w567 _ _ _ _ _ w751 w798]
          tunnel: [w508 w554 w603 w636 w669 w702 w735 w774 w821] -> w475
          tunnel: w478 -> [w491 w535 w579 w612 w645 w678 w711 w748 w797]
          tunnel: [w512 w557 w605 w638 w671 w704 w737 w776 w823] -> w477
          tunnel: [w516 w560 w608 w641 w674 w707 w740 w778 w825] -> w476
          tunnel: [w507 w553 w602 w635 w668 w701 w734 w773 w820] -> w474
          tunnel: [w506 w552 w601 w634 w667 w700 w733 w772 w819] -> w473
          tunnel: [w505 w551 w600 w633 w666 w699 w732 w771 w818] -> w472
          tunnel: [w504 w550 w599 w632 w665 w698 w731 w770 w817] -> w471
          tunnel: [w503 w549 w598 w631 w664 w697 w730 w769 w816] -> w470
          tunnel: [w502 w548 w597 w630 w663 w696 w729 w768 w815] -> w469
          tunnel: w468 -> [w515 w559 w607 w640 w673 w706 w739 w777 w824]
          tunnel: w467 -> [w511 w556 w604 w637 w670 w703 w736 w775 w822]
          tunnel: w466 -> [w499 w545 w594 w628 w661 w694 w727 w767 w814]
          tunnel: w465 -> [w498 w544 w593 w627 w660 w693 w726 w766 w813]
          tunnel: w464 -> [w497 w543 w592 w626 w659 w692 w725 w765 w812]
          tunnel: w463 -> [w496 w542 w591 w625 w658 w691 w724 w764 w811]
          tunnel: w462 -> [w495 w541 w590 w624 w657 w690 w723 w763 w810]
          tunnel: w461 -> [w494 w540 w589 w623 w656 w689 w722 w762 w809]
          tunnel: w460 -> [w493 w539 w588 w622 w655 w688 w721 w761 w808]
          tunnel: [w492 w536 w580 w613 w646 w679 w712 w745 w792] -> w459
          tunnel: w458 -> [w490 w534 w578 w611 w644 w677 w710 w744 w791]
          frame "mlight" {
            n244 = Index Array(array=w523, index=3) -> (element=w521:string)
            n245 = call <vilib>:"Trim Whitespace.vi"("string"=w521) -> ("trimmed string"=w520:string)  [unwired: 1 in]
            n246 = To Lower Case(string=w520) -> (all lower case string=w519:string)
            n247 = case shown="\"off\"" w519 {
              selector: w519 -> [_ w529 _]
              tunnel: w491 -> [w526 w530 w533]
              tunnel: [w525 w528 w532] -> w510
              frame "off" {
                w524 = 1
                n248 = local write "mlight"(w524) -> ()
                n249 = Bundle(w526, w524) -> (w525:cluster{timestamp, i32})  [unwired: 1 in]
              }
              frame Default {
                n250 = Decimal String To Number(string=w529) -> (number=w527:i32)  [unwired: 2 in, 1 out]
                n251 = local write "mlight"(w527) -> ()
                n252 = Bundle(w530, w527) -> (w528:cluster{timestamp, i32})  [unwired: 1 in]
              }
              frame "on" {
                w531 = 100
                n253 = local write "mlight"(w531) -> ()
                n254 = Bundle(w533, w531) -> (w532:cluster{timestamp, i32})  [unwired: 1 in]
              }
            }
            n255 = local read "plight"() -> (w518:i32)
            n256 = Bundle(w491, 0) -> (w501:cluster{timestamp, i32})  [unwired: 1 in]
            n257 = Bundle(w491, "plight"=w518) -> (w514:cluster{timestamp, "plight":i32})  [unwired: 1 in]
            n258 = Build Array(w514) -> (w513:cluster{timestamp, "plight":i32}[])
            n259 = Build Array(w501) -> (w500:cluster{timestamp, i32}[])
            n260 = Build Array(w510) -> (w509:cluster{timestamp, i32}[])
            n261 = Insert Into Array(array=w490, new element=w491) -> (w492:timestamp[])  [unwired: 1 in]
            n262 = Insert Into Array(array=w509, new element=w511) -> (w512:cluster{timestamp, i32}[])  [unwired: 1 in]
            n263 = Insert Into Array(array=w513, new element=w515) -> (w516:cluster{timestamp, "plight":i32}[])  [unwired: 1 in]
            n264 = Insert Into Array(array=w500, new element=w493) -> (w508:cluster{timestamp, i32}[])  [unwired: 1 in]
            n265 = Insert Into Array(array=w500, new element=w494) -> (w507:cluster{timestamp, i32}[])  [unwired: 1 in]
            n266 = Insert Into Array(array=w500, new element=w495) -> (w506:cluster{timestamp, i32}[])  [unwired: 1 in]
            n267 = Insert Into Array(array=w500, new element=w496) -> (w505:cluster{timestamp, i32}[])  [unwired: 1 in]
            n268 = Insert Into Array(array=w500, new element=w497) -> (w504:cluster{timestamp, i32}[])  [unwired: 1 in]
            n269 = Insert Into Array(array=w500, new element=w498) -> (w503:cluster{timestamp, i32}[])  [unwired: 1 in]
            n270 = Insert Into Array(array=w500, new element=w499) -> (w502:cluster{timestamp, i32}[])  [unwired: 1 in]
          }
          frame "plight" {
            n271 = Index Array(array=w567, index=3) -> (element=w565:string)
            n272 = call <vilib>:"Trim Whitespace.vi"("string"=w565) -> ("trimmed string"=w564:string)  [unwired: 1 in]
            n273 = To Lower Case(string=w564) -> (all lower case string=w563:string)
            n274 = case shown="\"on\"" w563 {
              selector: w563 -> [_ w573 _]
              tunnel: w535 -> [w570 w574 w577]
              tunnel: [w569 w572 w576] -> w555
              frame "off" {
                w568 = 1
                n275 = local write "plight"(w568) -> ()
                n276 = Bundle(w570, w568) -> (w569:cluster{timestamp, i32})  [unwired: 1 in]
              }
              frame Default {
                n277 = Decimal String To Number(string=w573) -> (number=w571:i32)  [unwired: 2 in, 1 out]
                n278 = local write "plight"(w571) -> ()
                n279 = Bundle(w574, w571) -> (w572:cluster{timestamp, i32})  [unwired: 1 in]
              }
              frame "on" {
                w575 = 100
                n280 = local write "plight"(w575) -> ()
                n281 = Bundle(w577, w575) -> (w576:cluster{timestamp, i32})  [unwired: 1 in]
              }
            }
            n282 = local read "mlight"() -> (w562:i32)
            n283 = Bundle(w535, 0) -> (w547:cluster{timestamp, i32})  [unwired: 1 in]
            n284 = Bundle(w535, "mlight"=w562) -> (w558:cluster{timestamp, "mlight":i32})  [unwired: 1 in]
            n285 = Build Array(w558) -> (w538:cluster{timestamp, "mlight":i32}[])
            n286 = Build Array(w547) -> (w546:cluster{timestamp, i32}[])
            n287 = Build Array(w555) -> (w537:cluster{timestamp, i32}[])
            n288 = Insert Into Array(array=w534, new element=w535) -> (w536:timestamp[])  [unwired: 1 in]
            n289 = Insert Into Array(array=w538, new element=w556) -> (w557:cluster{timestamp, "mlight":i32}[])  [unwired: 1 in]
            n290 = Insert Into Array(array=w537, new element=w559) -> (w560:cluster{timestamp, i32}[])  [unwired: 1 in]
            n291 = Insert Into Array(array=w546, new element=w539) -> (w554:cluster{timestamp, i32}[])  [unwired: 1 in]
            n292 = Insert Into Array(array=w546, new element=w540) -> (w553:cluster{timestamp, i32}[])  [unwired: 1 in]
            n293 = Insert Into Array(array=w546, new element=w541) -> (w552:cluster{timestamp, i32}[])  [unwired: 1 in]
            n294 = Insert Into Array(array=w546, new element=w542) -> (w551:cluster{timestamp, i32}[])  [unwired: 1 in]
            n295 = Insert Into Array(array=w546, new element=w543) -> (w550:cluster{timestamp, i32}[])  [unwired: 1 in]
            n296 = Insert Into Array(array=w546, new element=w544) -> (w549:cluster{timestamp, i32}[])  [unwired: 1 in]
            n297 = Insert Into Array(array=w546, new element=w545) -> (w548:cluster{timestamp, i32}[])  [unwired: 1 in]
          }
          frame "mpam", Default {
            n298 = local read "mlight"() -> (w610:i32)
            n299 = local read "plight"() -> (w585:i32)
            n300 = Bundle(w579, "mlight"=w610) -> (w606:cluster{timestamp, "mlight":i32})  [unwired: 1 in]
            n301 = Bundle(w579, "plight"=w585) -> (w583:cluster{timestamp, "plight":i32})  [unwired: 1 in]
            n302 = Bundle(w579, 0) -> (w596:cluster{timestamp, i32})  [unwired: 1 in]
            n303 = Bundle(w579, 70) -> (w582:cluster{timestamp, i32})  [unwired: 1 in]
            n304 = Build Array(w606) -> (w587:cluster{timestamp, "mlight":i32}[])
            n305 = Build Array(w583) -> (w586:cluster{timestamp, "plight":i32}[])
            n306 = Build Array(w596) -> (w595:cluster{timestamp, i32}[])
            n307 = Build Array(w582) -> (w581:cluster{timestamp, i32}[])
            n308 = Insert Into Array(array=w578, new element=w579) -> (w580:timestamp[])  [unwired: 1 in]
            n309 = Insert Into Array(array=w587, new element=w604) -> (w605:cluster{timestamp, "mlight":i32}[])  [unwired: 1 in]
            n310 = Insert Into Array(array=w586, new element=w607) -> (w608:cluster{timestamp, "plight":i32}[])  [unwired: 1 in]
            n311 = Insert Into Array(array=w581, new element=w588) -> (w603:cluster{timestamp, i32}[])  [unwired: 1 in]
            n312 = Insert Into Array(array=w595, new element=w589) -> (w602:cluster{timestamp, i32}[])  [unwired: 1 in]
            n313 = Insert Into Array(array=w595, new element=w590) -> (w601:cluster{timestamp, i32}[])  [unwired: 1 in]
            n314 = Insert Into Array(array=w595, new element=w591) -> (w600:cluster{timestamp, i32}[])  [unwired: 1 in]
            n315 = Insert Into Array(array=w595, new element=w592) -> (w599:cluster{timestamp, i32}[])  [unwired: 1 in]
            n316 = Insert Into Array(array=w595, new element=w593) -> (w598:cluster{timestamp, i32}[])  [unwired: 1 in]
            n317 = Insert Into Array(array=w595, new element=w594) -> (w597:cluster{timestamp, i32}[])  [unwired: 1 in]
          }
          frame "fstack" {
            n318 = local read "mlight"() -> (w643:i32)
            n319 = local read "plight"() -> (w619:i32)
            n320 = Bundle(w612, "mlight"=w643) -> (w639:cluster{timestamp, "mlight":i32})  [unwired: 1 in]
            n321 = Bundle(w612, "plight"=w619) -> (w617:cluster{timestamp, "plight":i32})  [unwired: 1 in]
            n322 = Bundle(w612, 0) -> (w629:cluster{timestamp, i32})  [unwired: 1 in]
            n323 = Bundle(w612, 40) -> (w616:cluster{timestamp, i32})  [unwired: 1 in]
            n324 = Build Array(w639) -> (w621:cluster{timestamp, "mlight":i32}[])
            n325 = Build Array(w617) -> (w620:cluster{timestamp, "plight":i32}[])
            n326 = Build Array(w629) -> (w615:cluster{timestamp, i32}[])
            n327 = Build Array(w616) -> (w614:cluster{timestamp, i32}[])
            n328 = Insert Into Array(array=w611, new element=w612) -> (w613:timestamp[])  [unwired: 1 in]
            n329 = Insert Into Array(array=w621, new element=w637) -> (w638:cluster{timestamp, "mlight":i32}[])  [unwired: 1 in]
            n330 = Insert Into Array(array=w620, new element=w640) -> (w641:cluster{timestamp, "plight":i32}[])  [unwired: 1 in]
            n331 = Insert Into Array(array=w615, new element=w622) -> (w636:cluster{timestamp, i32}[])  [unwired: 1 in]
            n332 = Insert Into Array(array=w614, new element=w623) -> (w635:cluster{timestamp, i32}[])  [unwired: 1 in]
            n333 = Insert Into Array(array=w615, new element=w624) -> (w634:cluster{timestamp, i32}[])  [unwired: 1 in]
            n334 = Insert Into Array(array=w615, new element=w625) -> (w633:cluster{timestamp, i32}[])  [unwired: 1 in]
            n335 = Insert Into Array(array=w615, new element=w626) -> (w632:cluster{timestamp, i32}[])  [unwired: 1 in]
            n336 = Insert Into Array(array=w615, new element=w627) -> (w631:cluster{timestamp, i32}[])  [unwired: 1 in]
            n337 = Insert Into Array(array=w615, new element=w628) -> (w630:cluster{timestamp, i32}[])  [unwired: 1 in]
          }
          frame "rfstack" {
            n338 = local read "mlight"() -> (w676:i32)
            n339 = local read "plight"() -> (w652:i32)
            n340 = Bundle(w645, "mlight"=w676) -> (w672:cluster{timestamp, "mlight":i32})  [unwired: 1 in]
            n341 = Bundle(w645, "plight"=w652) -> (w650:cluster{timestamp, "plight":i32})  [unwired: 1 in]
            n342 = Bundle(w645, 0) -> (w662:cluster{timestamp, i32})  [unwired: 1 in]
            n343 = Bundle(w645, 40) -> (w649:cluster{timestamp, i32})  [unwired: 1 in]
            n344 = Build Array(w672) -> (w654:cluster{timestamp, "mlight":i32}[])
            n345 = Build Array(w650) -> (w653:cluster{timestamp, "plight":i32}[])
            n346 = Build Array(w662) -> (w648:cluster{timestamp, i32}[])
            n347 = Build Array(w649) -> (w647:cluster{timestamp, i32}[])
            n348 = Insert Into Array(array=w644, new element=w645) -> (w646:timestamp[])  [unwired: 1 in]
            n349 = Insert Into Array(array=w654, new element=w670) -> (w671:cluster{timestamp, "mlight":i32}[])  [unwired: 1 in]
            n350 = Insert Into Array(array=w653, new element=w673) -> (w674:cluster{timestamp, "plight":i32}[])  [unwired: 1 in]
            n351 = Insert Into Array(array=w648, new element=w655) -> (w669:cluster{timestamp, i32}[])  [unwired: 1 in]
            n352 = Insert Into Array(array=w648, new element=w656) -> (w668:cluster{timestamp, i32}[])  [unwired: 1 in]
            n353 = Insert Into Array(array=w647, new element=w657) -> (w667:cluster{timestamp, i32}[])  [unwired: 1 in]
            n354 = Insert Into Array(array=w648, new element=w658) -> (w666:cluster{timestamp, i32}[])  [unwired: 1 in]
            n355 = Insert Into Array(array=w648, new element=w659) -> (w665:cluster{timestamp, i32}[])  [unwired: 1 in]
            n356 = Insert Into Array(array=w648, new element=w660) -> (w664:cluster{timestamp, i32}[])  [unwired: 1 in]
            n357 = Insert Into Array(array=w648, new element=w661) -> (w663:cluster{timestamp, i32}[])  [unwired: 1 in]
          }
          frame "rstack" {
            n358 = local read "mlight"() -> (w709:i32)
            n359 = local read "plight"() -> (w685:i32)
            n360 = Bundle(w678, "mlight"=w709) -> (w705:cluster{timestamp, "mlight":i32})  [unwired: 1 in]
            n361 = Bundle(w678, "plight"=w685) -> (w683:cluster{timestamp, "plight":i32})  [unwired: 1 in]
            n362 = Bundle(w678, 0) -> (w695:cluster{timestamp, i32})  [unwired: 1 in]
            n363 = Bundle(w678, 50) -> (w682:cluster{timestamp, i32})  [unwired: 1 in]
            n364 = Insert Into Array(array=w677, new element=w678) -> (w679:timestamp[])  [unwired: 1 in]
            n365 = Build Array(w705) -> (w687:cluster{timestamp, "mlight":i32}[])
            n366 = Build Array(w683) -> (w686:cluster{timestamp, "plight":i32}[])
            n367 = Build Array(w695) -> (w680:cluster{timestamp, i32}[])
            n368 = Build Array(w682) -> (w681:cluster{timestamp, i32}[])
            n369 = Insert Into Array(array=w687, new element=w703) -> (w704:cluster{timestamp, "mlight":i32}[])  [unwired: 1 in]
            n370 = Insert Into Array(array=w686, new element=w706) -> (w707:cluster{timestamp, "plight":i32}[])  [unwired: 1 in]
            n371 = Insert Into Array(array=w680, new element=w688) -> (w702:cluster{timestamp, i32}[])  [unwired: 1 in]
            n372 = Insert Into Array(array=w680, new element=w689) -> (w701:cluster{timestamp, i32}[])  [unwired: 1 in]
            n373 = Insert Into Array(array=w680, new element=w690) -> (w700:cluster{timestamp, i32}[])  [unwired: 1 in]
            n374 = Insert Into Array(array=w681, new element=w691) -> (w699:cluster{timestamp, i32}[])  [unwired: 1 in]
            n375 = Insert Into Array(array=w680, new element=w692) -> (w698:cluster{timestamp, i32}[])  [unwired: 1 in]
            n376 = Insert Into Array(array=w680, new element=w693) -> (w697:cluster{timestamp, i32}[])  [unwired: 1 in]
            n377 = Insert Into Array(array=w680, new element=w694) -> (w696:cluster{timestamp, i32}[])  [unwired: 1 in]
          }
          frame "stack" {
            n378 = local read "mlight"() -> (w742:i32)
            n379 = local read "plight"() -> (w718:i32)
            n380 = Bundle(w711, "mlight"=w742) -> (w738:cluster{timestamp, "mlight":i32})  [unwired: 1 in]
            n381 = Bundle(w711, "plight"=w718) -> (w716:cluster{timestamp, "plight":i32})  [unwired: 1 in]
            n382 = Bundle(w711, 0) -> (w728:cluster{timestamp, i32})  [unwired: 1 in]
            n383 = Bundle(w711, 50) -> (w715:cluster{timestamp, i32})  [unwired: 1 in]
            n384 = Build Array(w738) -> (w720:cluster{timestamp, "mlight":i32}[])
            n385 = Build Array(w716) -> (w719:cluster{timestamp, "plight":i32}[])
            n386 = Build Array(w728) -> (w714:cluster{timestamp, i32}[])
            n387 = Build Array(w715) -> (w713:cluster{timestamp, i32}[])
            n388 = Insert Into Array(array=w710, new element=w711) -> (w712:timestamp[])  [unwired: 1 in]
            n389 = Insert Into Array(array=w720, new element=w736) -> (w737:cluster{timestamp, "mlight":i32}[])  [unwired: 1 in]
            n390 = Insert Into Array(array=w719, new element=w739) -> (w740:cluster{timestamp, "plight":i32}[])  [unwired: 1 in]
            n391 = Insert Into Array(array=w714, new element=w721) -> (w735:cluster{timestamp, i32}[])  [unwired: 1 in]
            n392 = Insert Into Array(array=w714, new element=w722) -> (w734:cluster{timestamp, i32}[])  [unwired: 1 in]
            n393 = Insert Into Array(array=w714, new element=w723) -> (w733:cluster{timestamp, i32}[])  [unwired: 1 in]
            n394 = Insert Into Array(array=w714, new element=w724) -> (w732:cluster{timestamp, i32}[])  [unwired: 1 in]
            n395 = Insert Into Array(array=w713, new element=w725) -> (w731:cluster{timestamp, i32}[])  [unwired: 1 in]
            n396 = Insert Into Array(array=w714, new element=w726) -> (w730:cluster{timestamp, i32}[])  [unwired: 1 in]
            n397 = Insert Into Array(array=w714, new element=w727) -> (w729:cluster{timestamp, i32}[])  [unwired: 1 in]
          }
          frame "rscan" {
            n398 = Index Array(array=w751, index=4) -> (element=w757:string)
            n399 = Index Array(array=w751, index=3) -> (element=w759:string)
            n400 = Fract/Exp String To Number(string=w759) -> (number=w755:dbl)  [unwired: 3 in, 1 out]
            n401 = Fract/Exp String To Number(string=w757) -> (number=w756:dbl)  [unwired: 3 in, 1 out]
            n402 = Equal To 0?(x=w755) -> (x = 0?=w754:bool)
            n403 = Select(t=1.0, s=w754, f=w755) -> (s? t:f=w752:dbl)
            n404 = for {
              N: w752 -> [_]
              tunnel: [w789] -> w749 mode=indexing
              tunnel: w756 -> [w788]
              shift-right: [w779] -> _
              shift-left: w748 -> [w787]
              tunnel: [w786] -> w750 mode=indexing
              tunnel: [w782] -> w747 mode=indexing
              tunnel: [w781] -> w746 mode=indexing
              tunnel: [w779] -> w743 mode=indexing
              n405 = local read "mlight"() -> (w783:i32)
              n406 = local read "plight"() -> (w784:i32)
              n407 = Add(x=w787, y=w788) -> (x+y=w779:timestamp)
              n408 = Bundle(w779, 50) -> (w789:cluster{timestamp, i32})  [unwired: 1 in]
              n409 = Bundle(w779, 0) -> (w786:cluster{timestamp, i32})  [unwired: 1 in]
              n410 = Bundle(w779, "mlight"=w783) -> (w782:cluster{timestamp, "mlight":i32})  [unwired: 1 in]
              n411 = Bundle(w779, "plight"=w784) -> (w781:cluster{timestamp, "plight":i32})  [unwired: 1 in]
            }
            n412 = Insert Into Array(array=w747, new element=w775) -> (w776:cluster{timestamp, "mlight":i32}[])  [unwired: 1 in]
            n413 = Insert Into Array(array=w746, new element=w777) -> (w778:cluster{timestamp, "plight":i32}[])  [unwired: 1 in]
            n414 = Insert Into Array(array=w750, new element=w761) -> (w774:cluster{timestamp, i32}[])  [unwired: 1 in]
            n415 = Insert Into Array(array=w750, new element=w762) -> (w773:cluster{timestamp, i32}[])  [unwired: 1 in]
            n416 = Insert Into Array(array=w750, new element=w763) -> (w772:cluster{timestamp, i32}[])  [unwired: 1 in]
            n417 = Insert Into Array(array=w750, new element=w764) -> (w771:cluster{timestamp, i32}[])  [unwired: 1 in]
            n418 = Insert Into Array(array=w750, new element=w765) -> (w770:cluster{timestamp, i32}[])  [unwired: 1 in]
            n419 = Insert Into Array(array=w749, new element=w766) -> (w769:cluster{timestamp, i32}[])  [unwired: 1 in]
            n420 = Insert Into Array(array=w750, new element=w767) -> (w768:cluster{timestamp, i32}[])  [unwired: 1 in]
            n421 = Insert Into Array(array=w743, new element=w744) -> (w745:timestamp[])  [unwired: 1 in]
          }
          frame "scan" {
            n422 = Index Array(array=w798, index=4) -> (element=w804:string)
            n423 = Index Array(array=w798, index=3) -> (element=w806:string)
            n424 = Fract/Exp String To Number(string=w806) -> (number=w802:dbl)  [unwired: 3 in, 1 out]
            n425 = Fract/Exp String To Number(string=w804) -> (number=w803:dbl)  [unwired: 3 in, 1 out]
            n426 = Equal To 0?(x=w802) -> (x = 0?=w801:bool)
            n427 = Select(t=1.0, s=w801, f=w802) -> (s? t:f=w799:dbl)
            n428 = for {
              N: w799 -> [_]
              tunnel: [w836] -> w794 mode=indexing
              tunnel: w803 -> [w835]
              shift-right: [w826] -> _
              shift-left: w797 -> [w834]
              tunnel: [w833] -> w793 mode=indexing
              tunnel: [w829] -> w796 mode=indexing
              tunnel: [w828] -> w795 mode=indexing
              tunnel: [w826] -> w790 mode=indexing
              n429 = local read "mlight"() -> (w830:i32)
              n430 = local read "plight"() -> (w831:i32)
              n431 = Add(x=w834, y=w835) -> (x+y=w826:timestamp)
              n432 = Bundle(w826, 60) -> (w836:cluster{timestamp, i32})  [unwired: 1 in]
              n433 = Bundle(w826, 0) -> (w833:cluster{timestamp, i32})  [unwired: 1 in]
              n434 = Bundle(w826, "mlight"=w830) -> (w829:cluster{timestamp, "mlight":i32})  [unwired: 1 in]
              n435 = Bundle(w826, "plight"=w831) -> (w828:cluster{timestamp, "plight":i32})  [unwired: 1 in]
            }
            n436 = Insert Into Array(array=w790, new element=w791) -> (w792:timestamp[])  [unwired: 1 in]
            n437 = Insert Into Array(array=w796, new element=w822) -> (w823:cluster{timestamp, "mlight":i32}[])  [unwired: 1 in]
            n438 = Insert Into Array(array=w795, new element=w824) -> (w825:cluster{timestamp, "plight":i32}[])  [unwired: 1 in]
            n439 = Insert Into Array(array=w793, new element=w808) -> (w821:cluster{timestamp, i32}[])  [unwired: 1 in]
            n440 = Insert Into Array(array=w793, new element=w809) -> (w820:cluster{timestamp, i32}[])  [unwired: 1 in]
            n441 = Insert Into Array(array=w793, new element=w810) -> (w819:cluster{timestamp, i32}[])  [unwired: 1 in]
            n442 = Insert Into Array(array=w793, new element=w811) -> (w818:cluster{timestamp, i32}[])  [unwired: 1 in]
            n443 = Insert Into Array(array=w793, new element=w812) -> (w817:cluster{timestamp, i32}[])  [unwired: 1 in]
            n444 = Insert Into Array(array=w793, new element=w813) -> (w816:cluster{timestamp, i32}[])  [unwired: 1 in]
            n445 = Insert Into Array(array=w794, new element=w814) -> (w815:cluster{timestamp, i32}[])  [unwired: 1 in]
          }
        }
        "strip array 3" <- w479
      }
      n446 = Build Cluster Array(w448, w457, w456, w455, w454, w453, w452, w451, w450) -> (w447:cluster{cluster{timestamp, dbl}[]}[])
    }
  }
  "timer graph" <- w12
  "time array" <- w10
  "array of clusters 2" <- w12
  "settings array out" <- w1
  n447 = Array Max & Min(array=w10) -> (max value=w25:timestamp, min value=w24:timestamp)  [unwired: 2 out]
  n448 = Get Date/Time In Seconds() -> (seconds since 1Jan1904=w23:timestamp)
  n449 = To Double Precision Float(number=w25) -> (double precision float=w21:dbl)
  n450 = To Double Precision Float(number=w23) -> (double precision float=w20:dbl)
  "cursor position" <- w20
  n451 = Max & Min(x=w24, y=w23) -> (min(x,y)=w22:timestamp)  [unwired: 1 out]
  n452 = To Double Precision Float(number=w22) -> (double precision float=w17:dbl)
  n453 = Subtract(x=w21, y=w17) -> (x-y=w19:dbl)
  n454 = Divide(x=w19, y=50.0) -> (x/y=w14:dbl)
  n455 = Add(x=w21, y=w14) -> (x+y=w15:dbl)
  "Xscalemax" <- w15
  n456 = Subtract(x=w17, y=w14) -> (x-y=w16:dbl)
  "Xscle min" <- w16
  n457 = property on="timer graph" class="XYGraph (strict)"("Cursor.Cursor X"=w20, "XScale.Minimum"=w16, "XScale.Maximum"=w15) -> ()  [unwired: 2 in, 2 out]
